vi "Covert Max &Min data in String.vi"() -> (3 "out":T1)   [LabVIEW 2015]
uses:
  Galobal variable_TI.vi
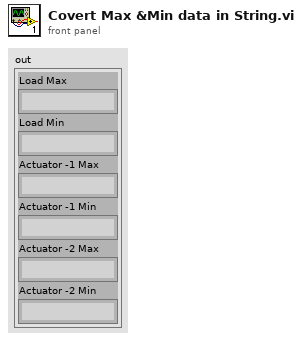
[diagram p1: front panel]
types:
  T1 = cluster{"Load Max":string, "Load Min":string, "Actuator -1 Max":string, "Actuator -1 Min":string, "Actuator -2 Max":string, "Actuator -2 Min":string}
  T2 = cluster{"Load Max(N)":dbl, "Load Min(N)":dbl, "Actuator1 max(mm)":dbl, "Actuator1min(mm)":dbl, "Actuator2 max(mm)":dbl, "Actuator2min(mm)":dbl, "Load Offset":dbl, "Model":string, "MIC Code":string}
  T3 = cluster{"[0]":string, "[1]":string, "[2]":string, "[3]":string, "[4]":string, "[5]":string}
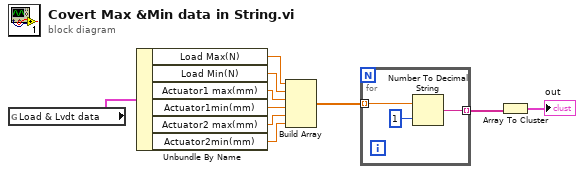
[diagram p0: block diagram]
diagram:
  n1 = global read "Galobal variable_TI.vi" "Load & Lvdt data"() -> (w10:T2)
  n2 = Unbundle By Name(w10) -> ("Load Max(N)"=w9:dbl, "Load Min(N)"=w8:dbl, "Actuator1 max(mm)"=w7:dbl, "Actuator1min(mm)"=w6:dbl, "Actuator2 max(mm)"=w5:dbl, "Actuator2min(mm)"=w4:dbl)
  n3 = Build Array(w9, w8, w7, w6, w5, w4) -> (w3:dbl[])
  n4 = for {
    tunnel: w3 -> [w12] mode=indexing
    tunnel: [w11] -> w2 mode=indexing
    n5 = Number To Decimal String(number=w12, width (-)=i16 1) -> (decimal integer string=w11:string)
  }
  n6 = Array To Cluster(array=w2) -> (cluster=→"out":T3)
